vi "SDO_TRAJECTORY_CALC_ORIENTATION.vi"(0 "Time Period":dbl=0.02, 4 "Starting Fraction":dbl=0.1, 6 "Completion Fraction":dbl=0.8, 8 "Init":bool, 9 "Time Fraction":dbl, 10 "End Orientation Demand DEG":dbl, 11 "Starting Orientation":T1 {"SIN" format="%13.4f"; "COS" format="%13.4f"; "VALUE" format="%13.4f"}) -> (1 "Rotational Velocity":dbl, 2 "Orientation Demand Deg":dbl, 3 "Orientation Demand":T1 {"SIN" format="%13.4f"; "COS" format="%13.4f"; "VALUE" format="%13.4f"})   [LabVIEW 2019]
uses:
  <vilib>/Rock Robotics/WPI/ThirdParty/JAS_Junk/TrajLib/TypeDef/ROTATION2D.ctl
  <vilib>/Rock Robotics/WPI/ThirdParty/JAS_Junk/TrajLib/Conv_Deg_Radians.vi
  <vilib>/Rock Robotics/WPI/ThirdParty/JAS_Junk/TrajLib/Rotation2d_CreateAngle.vi
  <vilib>/Rock Robotics/WPI/ThirdParty/JAS_Junk/TrajLib/Rotation2d_Plus.vi
  <vilib>/Rock Robotics/WPI/ThirdParty/JAS_Junk/TrajLib/Rotation2d_Minus.vi
  <vilib>/Rock Robotics/WPI/ThirdParty/JAS_Junk/TrajLib/MathUtil_Clamp.vi
  <vilib>/Rock Robotics/WPI/ThirdParty/JAS_Junk/TrajLib/Rotation2d_Times.vi
  <vilib>/Rock Robotics/WPI/ThirdParty/JAS_Junk/TrajLib/MathUtil_InputModulus.vi
  <vilib>/Rock Robotics/WPI/ThirdParty/JAS_Junk/TrajLib/Rotation2d_GetRadians.vi
  <vilib>/Rock Robotics/WPI/ThirdParty/JAS_Junk/TrajLib/Conv_Radians_Deg.vi
  <vilib>/Rock Robotics/WPI/ThirdParty/JAS_Junk/TrajLib/Rotation2d_RotateBy.vi
  <vilib>/Rock Robotics/WPI/ThirdParty/JAS_Junk/TrajLib/Rotation2d_UnaryMinus.vi
  <vilib>/Rock Robotics/WPI/ThirdParty/JAS_Junk/TrajLib/Rotation2d_CreateXY.vi
  <vilib>/Rock Robotics/WPI/ThirdParty/JAS_Junk/TrajLib/Util_CalcDist.vi
  <vilib>/Rock Robotics/WPI/ThirdParty/JAS_Junk/TrajLib/Trajectory_Library.lvlib
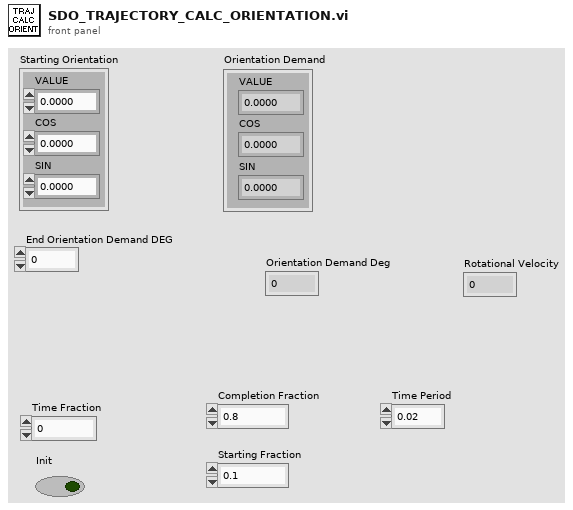
[diagram p1: front panel]
types:
  T1 = typedef "Trajectory_Library.lvlib/ROTATION2D.ctl" = cluster{"VALUE":dbl, "COS":dbl, "SIN":dbl}
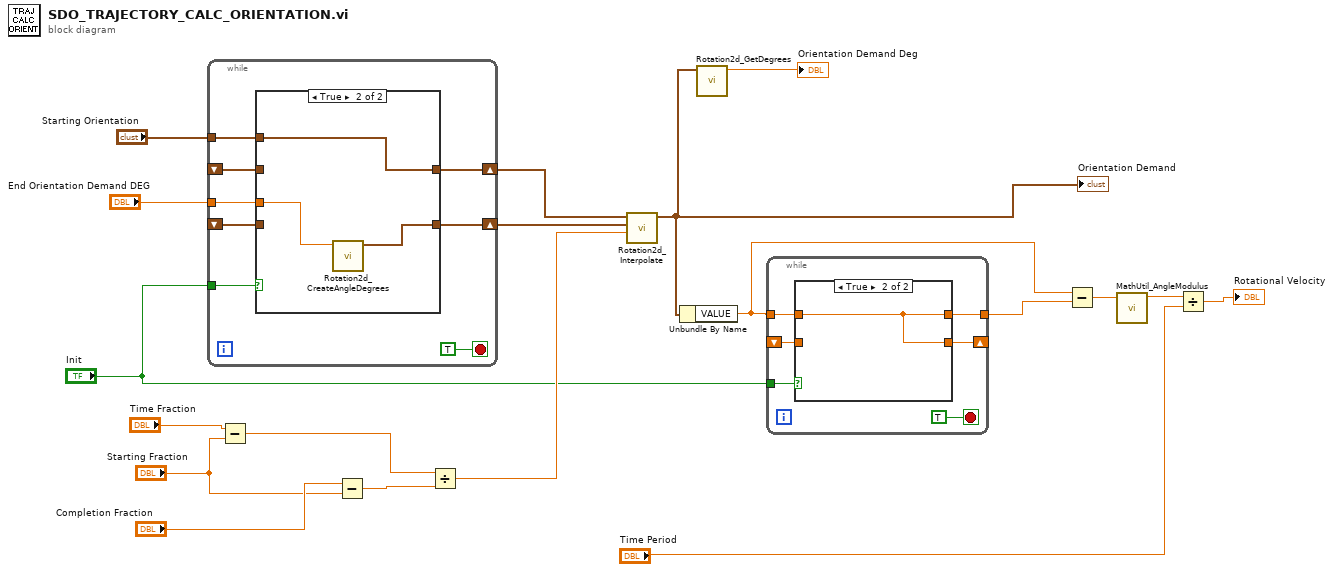
[diagram p0: block diagram]
diagram:
  n1 = while {
    tunnel: "Init" -> [w26]
    tunnel: "Starting Orientation" -> [w25]
    tunnel: "End Orientation Demand DEG" -> [w24]
    shift-right: [w22] -> w14
    shift-left: _ -> [w20]
    shift-right: [w23] -> w17
    shift-left: _ -> [w21]
    stop <- TRUE stop-if-true
    n2 = case shown="True" w26 {
      tunnel: w25 -> [_ w31]
      tunnel: w24 -> [_ w32]
      tunnel: [w29 w31] -> w23
      tunnel: [w28 w30] -> w22
      tunnel: w21 -> [w29 _]
      tunnel: w20 -> [w28 _]
      frame False {
      }
      frame True {
        n3 = call <vilib>:"Rotation2d_CreateAngleDegrees.vi"("Angle_Degrees"=w32) -> ("ROTATION"=w30:T1)  [unwired: 10 in]
      }
    }
  }
  n4 = Subtract(x="Time Fraction", y="Starting Fraction") -> (x-y=w9:dbl)
  n5 = Subtract(x="Completion Fraction", y="Starting Fraction") -> (x-y=w10:dbl)
  n6 = Divide(x=w9, y=w10) -> (x/y=w16:dbl)
  n7 = call <vilib>:"Rotation2d_Interpolate.vi"("T"=w16, "EncValue ROTATION"=w14, "in ROTATION"=w17) -> ("Interpolated ROTATION"=w7:T1)  [unwired: 8 in]
  "Orientation Demand" <- w7
  n8 = Unbundle By Name(w7) -> ("VALUE"=w6:dbl)
  n9 = call <vilib>:"Rotation2d_GetDegrees.vi"("in ROTATION"=w7) -> ("AngleDegrees"=→"Orientation Demand Deg":dbl)  [unwired: 10 in]
  n10 = while {
    tunnel: "Init" -> [w37]
    tunnel: w6 -> [w36]
    shift-right: [w35] -> _
    shift-left: _ -> [w34]
    tunnel: [w33] -> w1
    stop <- TRUE stop-if-true
    n11 = case shown="True" w37 {
      tunnel: w36 -> [w39 w41]
      tunnel: [w39 w41] -> w35
      tunnel: w34 -> [w40 _]
      tunnel: [w40 w41] -> w33
      frame False {
      }
      frame True {
      }
    }
  }
  n12 = Subtract(x=w6, y=w1) -> (x-y=w5:dbl)
  n13 = call <vilib>:"MathUtil_AngleModulus.vi"("InputAngle"=w5) -> ("ModulsAngle"=w4:dbl)  [unwired: 10 in]
  n14 = Divide(x=w4, y="Time Period") -> (x/y=→"Rotational Velocity":dbl)
